vi "Lights Immediate.vi"(7 "Description":string, 8 "Command Info In":T1, 9 "Speed":dbl, 10 "Flash Type":dbl, 11 "Color":dbl) -> (0 "Command Info Out":T1)   [LabVIEW 2020]
doc: "This template is useful for immediate subsystem actions that do not need deadband filtering\n\nBe sure to right-click and select New from Template and save with a new command name."
uses:
  <vilib>/Rock Robotics/WPI/Framework/Command Status Info.ctl
  <vilib>/Rock Robotics/WPI/Framework/Completion Status.ctl
  <vilib>/Rock Robotics/WPI/Framework/Completion Notifier.ctl
  Implementation/Lights Setpoints.ctl
  Implementation/Lights Operations.ctl
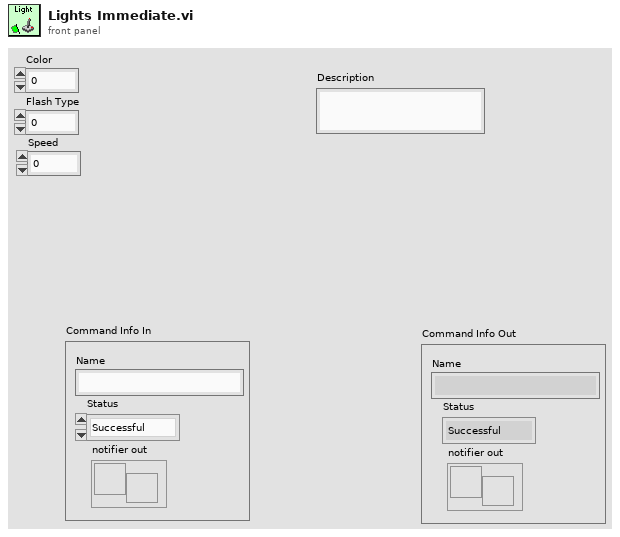
[diagram p1: front panel]
types:
  T1 = typedef "Command Status Info.ctl" = cluster{"Name":string, "Status":T2, "notifier out":T3}
  T2 = typedef "Completion Status.ctl" = enum16{"Successful", "Aborted", "Incomplete"}
  T3 = typedef "Completion Notifier.ctl" = refnum<notifier>
  T4 = typedef "Lights Setpoints.ctl" = cluster{"Operation":T5, "Color":dbl, "Flash Type":dbl, "Speed":dbl}
  T5 = typedef "Lights Operations.ctl" = enum16{"Reserve", "Read Current", "Immediate"}
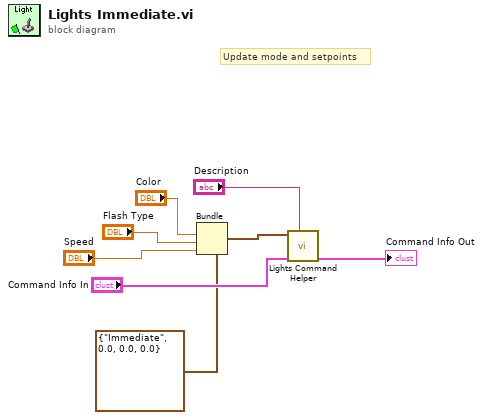
[diagram p0: block diagram]
diagram:
  # "Update mode and setpoints"
  n1 = Bundle(cluster=T4 {"Operation"=enum."Immediate", "Color"=0.0, "Flash Type"=0.0, "Speed"=0.0} ("SubSystem Data"), "Color"="Color", "Flash Type"="Flash Type", "Speed"="Speed") -> (w4:T4)  [unwired: 1 in]
  n2 = call "Lights Command Helper.vi"("Description"="Description", "Command Info In"="Command Info In", "SubSystem Data"=w4) -> ("Command Info Out"=→"Command Info Out":T1)  [unwired: 6 in, 2 out]
